vi "Clean Up Children.vi"(8 "error in (no error)":errorcluster, 9 "Folder Names":string[](array[string]), 10 "Parent Tag":string, 11 "Tree In":refnum<vi>) -> (0 "error out":errorcluster, 1 "Folder Names Dup":string[](array[string]), 2 "Parent Tag Dup":string, 3 "Tree Out":refnum<vi>)   [LabVIEW 2018, in "Tree Browser.lvlib"]
doc: "Deletes any children immediately under a parent node which don't exist on disk."
uses:
  Tree Browser.lvlib
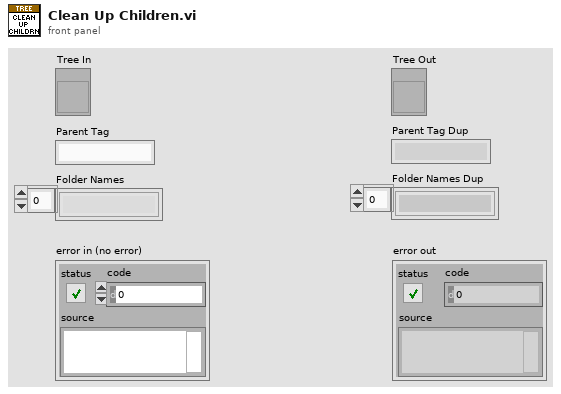
[diagram p1: front panel]
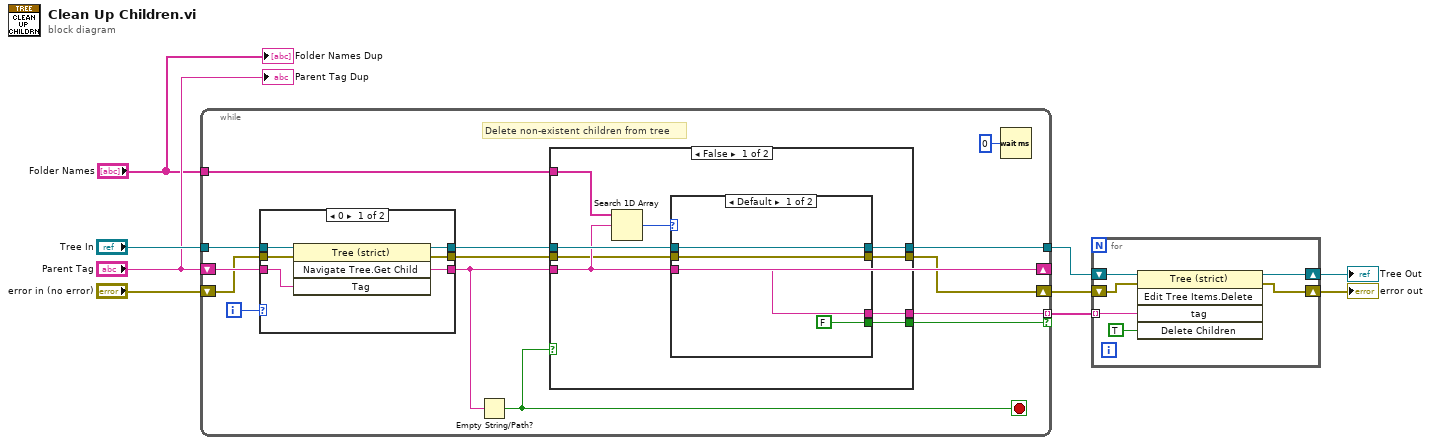
[diagram p0: block diagram]
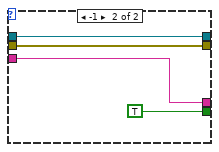
[diagram p2: hidden frame]
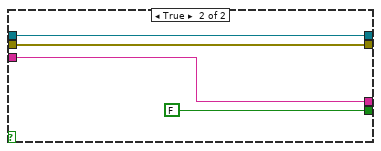
[diagram p3: hidden frame]
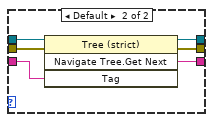
[diagram p4: hidden frame]
diagram:
  n1 = while {
    tunnel: "Tree In" -> [w23]
    shift-right: [w19] -> _
    shift-left: "Parent Tag" -> [w21]
    tunnel: "Folder Names" -> [w17]
    tunnel: [w16] -> w4
    shift-right: [w13] -> w2
    shift-left: "error in (no error)" -> [w15]
    tunnel: [w12] -> w5 mode=indexing if=w11
    i -> [w22]
    stop <- w20 stop-if-true
    # "Delete non-existent children from tree"
    n2 = case shown="0" w22 {
      tunnel: w23 -> [w50 w56]
      tunnel: w21 -> [w49 w51]
      tunnel: [w48 w55] -> w19
      tunnel: [w47 w54] -> w18
      tunnel: w15 -> [w46 w53]
      tunnel: [w45 w52] -> w14
      frame 0 {
        n3 = invoke class="Tree (strict)" method="Navigate Tree.Get Child"(reference=w50, error in=w46, "Tag"=w49) -> (reference out=w47:refnum<vi>, error out=w45:errorcluster, "Navigate Tree:Get Child"=w48:string)  [unwired: 1 in, 1 out]
      }
      frame Default {
        n4 = invoke class="Tree (strict)" method="Navigate Tree.Get Next"(reference=w56, error in=w53, "Tag"=w51) -> (reference out=w54:refnum<vi>, error out=w52:errorcluster, "Navigate Tree:Get Next Item"=w55:string)  [unwired: 1 in, 1 out]
      }
    }
    n5 = Empty String/Path?(string/path=w19) -> (empty?=w20:bool)
    n6 = case shown="False" w20 {
      tunnel: w18 -> [w31 w44]
      tunnel: w17 -> [w30 _]
      tunnel: w19 -> [w29 w42]
      tunnel: [w28 w44] -> w16
      tunnel: w14 -> [w27 w43]
      tunnel: [w26 w43] -> w13
      tunnel: [w25 w42] -> w12
      tunnel: [w24 FALSE] -> w11
      frame False {
        n7 = Search 1D Array(1D array=w30, element=w29) -> (index of element=w32:i32)  [unwired: 1 in]
        n8 = case shown="Default" w32 {
          tunnel: w31 -> [w36 w39]
          tunnel: w29 -> [w34 w40]
          tunnel: [w36 w39] -> w28
          tunnel: w27 -> [w35 w38]
          tunnel: [w35 w38] -> w26
          tunnel: [w34 w40] -> w25
          tunnel: [FALSE TRUE] -> w24
          frame Default {
          }
          frame -1 {
          }
        }
      }
      frame True {
      }
    }
    n9 = Wait (ms)(milliseconds to wait=u32 0) -> ()  [unwired: 1 out]
  }
  n10 = for {
    tunnel: w5 -> [w61] mode=indexing
    shift-right: [w57] -> w1
    shift-left: w2 -> [w58]
    shift-right: [w59] -> w3
    shift-left: w4 -> [w60]
    n11 = invoke class="Tree (strict)" method="Edit Tree Items.Delete"(reference=w60, error in=w58, "tag"=w61, "Delete Children"=TRUE ("Delete Children?")) -> (reference out=w59:refnum<vi>, error out=w57:errorcluster)  [unwired: 1 in, 3 out]
  }
  "Tree Out" <- w3
  "error out" <- w1
  "Parent Tag Dup" <- "Parent Tag"
  "Folder Names Dup" <- "Folder Names"
